vi "Timer.vi"(1 "Reset Timer":bool) -> (0 "Time (ms)":u32)   [LabVIEW 2019]
doc: "This VI runs a relative millisecond timer. Setting Reset Timer to TRUE will reset the timer to 0 ms."
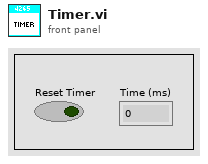
[diagram p1: front panel]
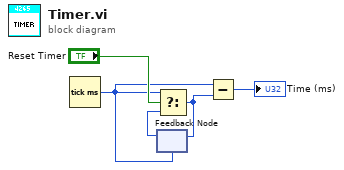
[diagram p0: block diagram]
diagram:
  n1 = Tick Count (ms)() -> (millisecond timer value=w2:u32)
  n2 = feedback #1(w2) -> (w1:u32)
  n3 = Select(t=w2, s="Reset Timer", f=w1) -> (s? t:f=w3:u32)
  n4 = feedback-in #1(w3) -> ()
  n5 = Subtract(x=w2, y=w3) -> (x-y=→"Time (ms)":u32)
